vi "Main.vi"(11 "error in (no error)":errorcluster) -> (15 "error out":errorcluster)   [LabVIEW 2023]
uses:
  Controls/Operation.ctl
  Controls/State Cluster.ctl
  Controls/Main Data Cluster.ctl
  Controls/Sender Clone Cluster.ctl
  Controls/Receiver Clone Cluster.ctl
  Classes/Receiver/Receiver UI.vi
  Classes/Sender/Sender UI.vi
  Classes/Receiver/Receiver.lvclass
  Classes/Sender/Sender.lvclass
panel:
  in  "Receiver Clones":string(combo)
  in  "Sender Clones":string(combo)
  in  "Create Receiver Clone":bool
  in  "Create Sender Clone":bool
  in  "Load Receiver":bool
  in  "Load Sender":bool
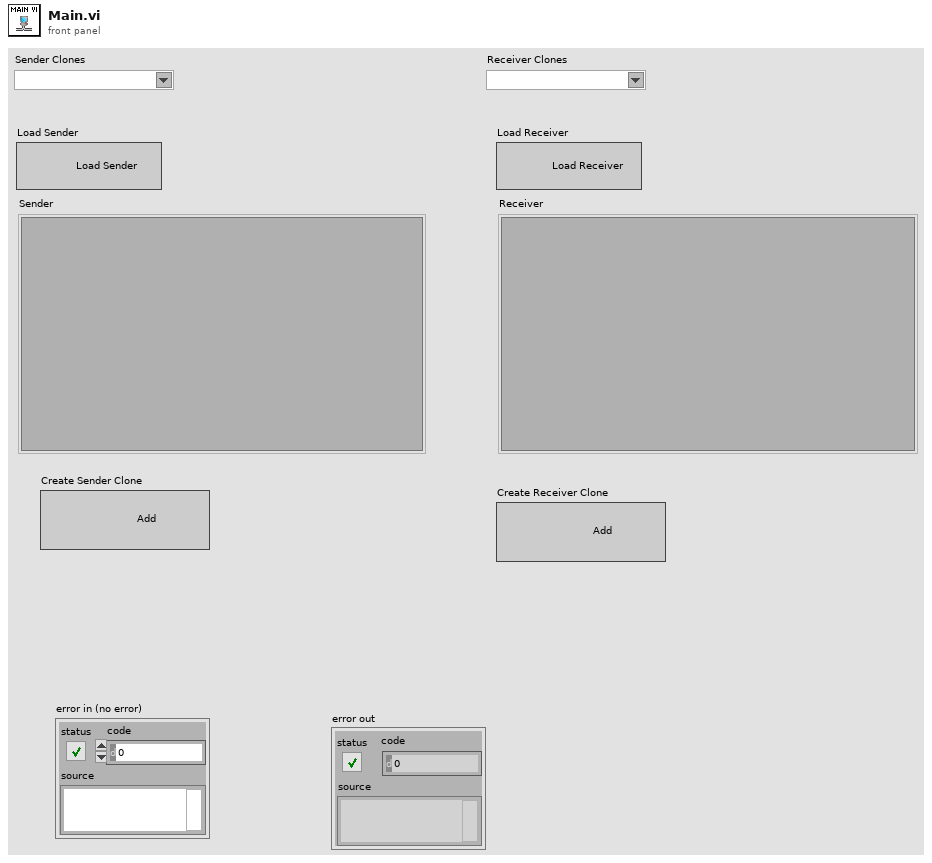
[diagram p1: front panel]
types:
  T1 = typedef "Main Data Cluster.ctl" = cluster{"user event out":refnum<user-event>, "Sender Path":path, "Receiver Path":path, "Sender Name":string, "Receiver Name":string, "Sender Combo Box":string[], "Sender Clone Data":T2[], "Receiver Clone Data":T3[], "Receiver Combo Box":string[], "Selected Receiver Clone":string, "Selected Sender Clone":string, "Sender VI Refnum":refnum<vi>, "Receiver VI Refnum":refnum<vi>, "Load/Unload Sender":bool, "Load/Unload Receiver":bool}
  T2 = typedef "Sender Clone Cluster.ctl" = cluster{"Sender Clone Name":string, "Sender VI reference":refnum<vi>}
  T3 = typedef "Receiver Clone Cluster.ctl" = cluster{"Receiver Clone Name":string, "Receiver VI Reference":refnum<vi>}
  T4 = typedef "State Cluster.ctl" = cluster{"State":string, "Data":variant}
  T5 = typedef "Operation.ctl" = enum16{"Create", "Enqueue", "Enqueue N", "Enstack", "Dequeue", "Flush", "Release"}
  T6 = enum8{"Enabled", "Disabled", "Disabled and Grayed Out"}
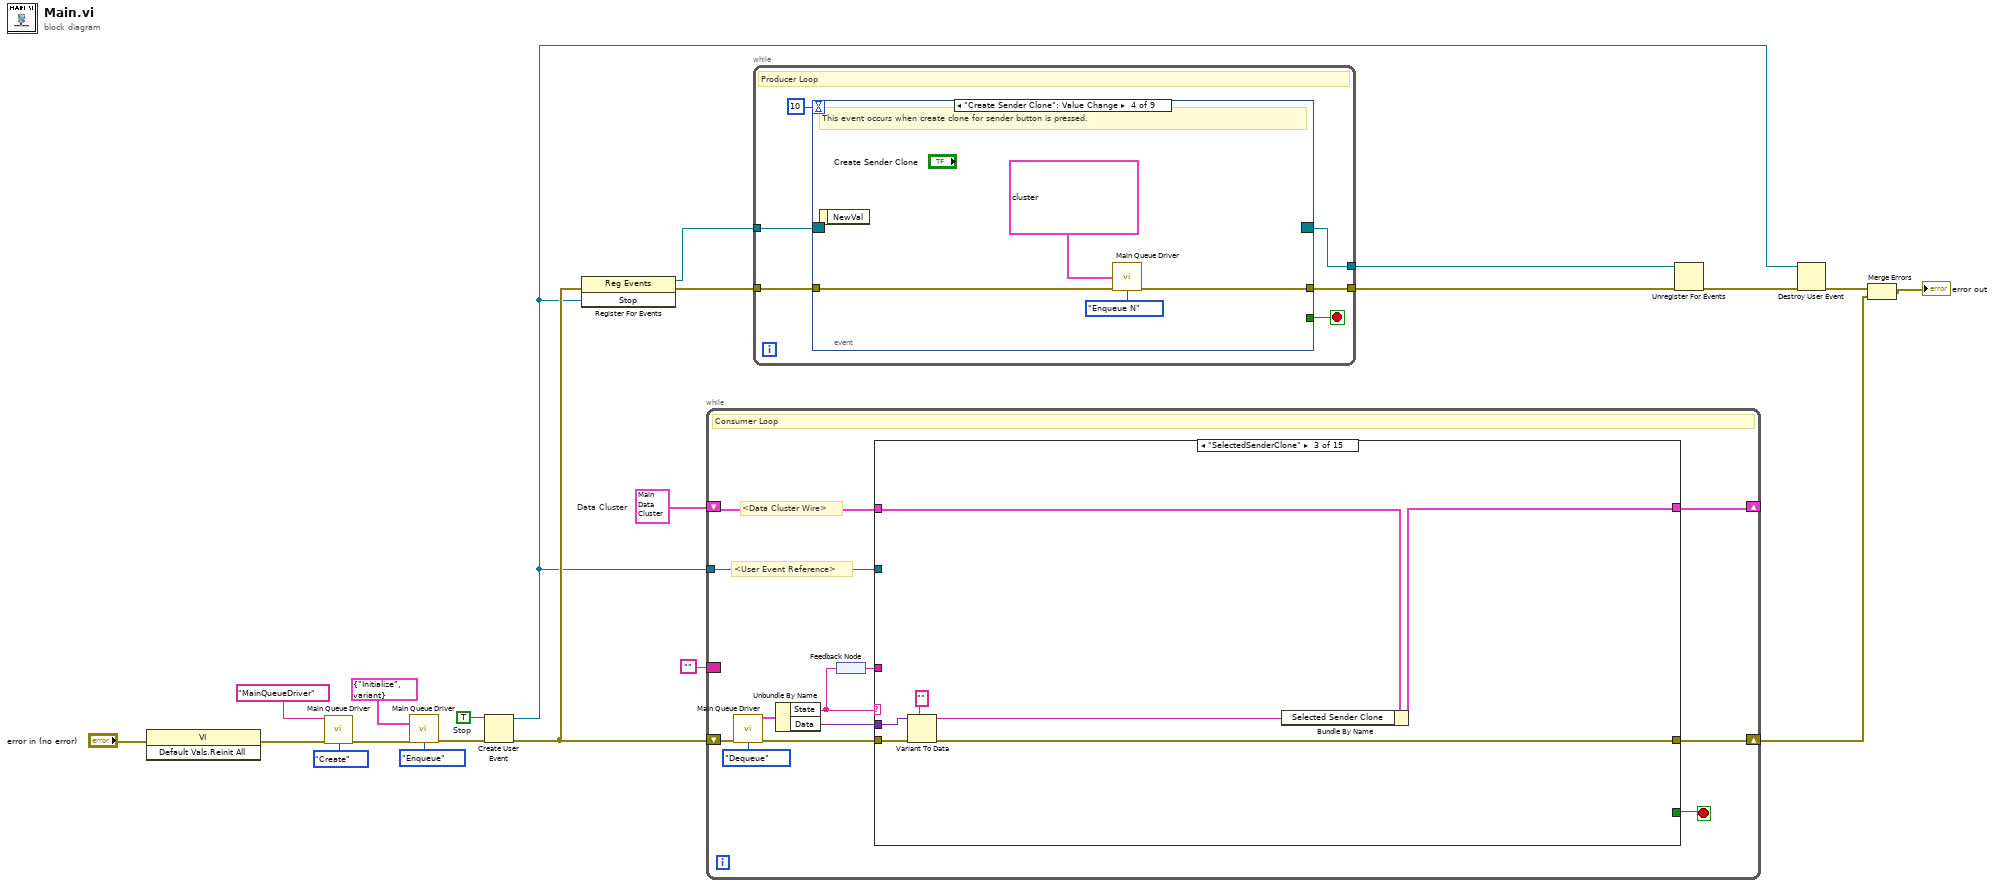
[diagram p0: block diagram]
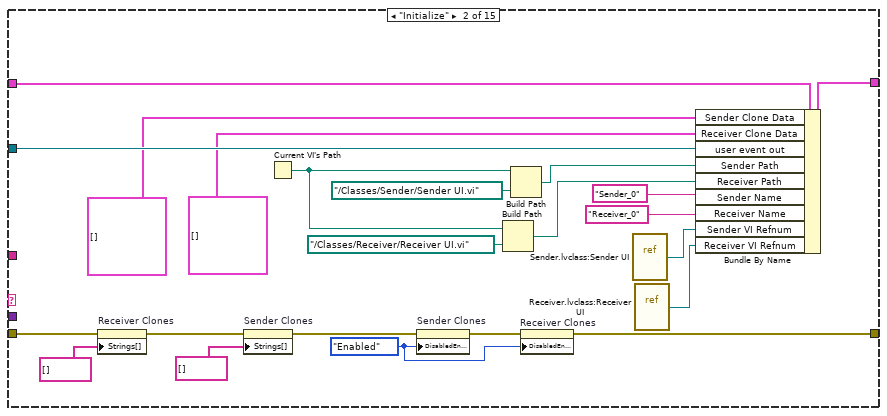
[diagram p3: hidden frame]
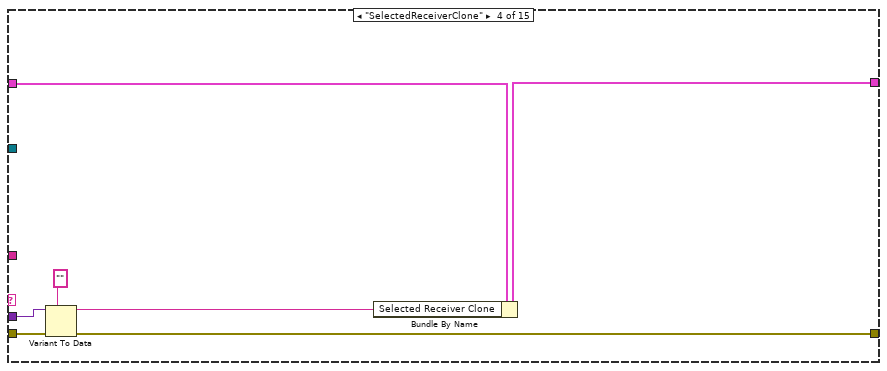
[diagram p4: hidden frame]
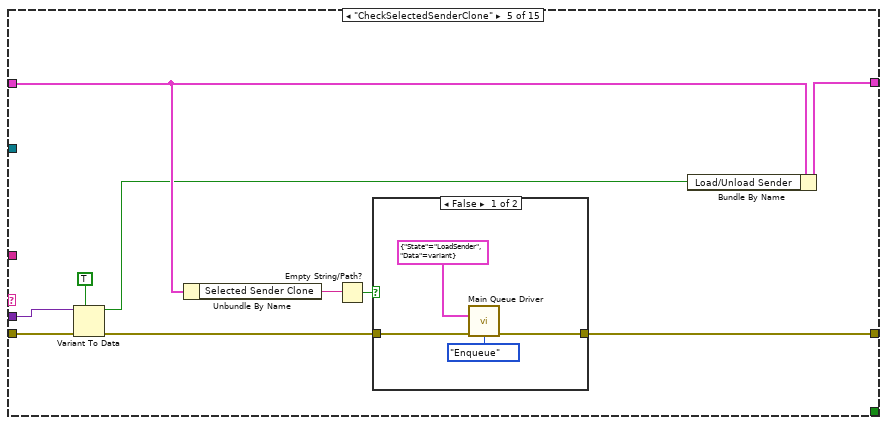
[diagram p5: hidden frame]
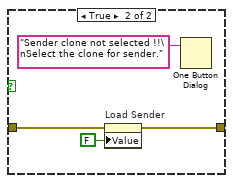
[diagram p6: hidden frame]
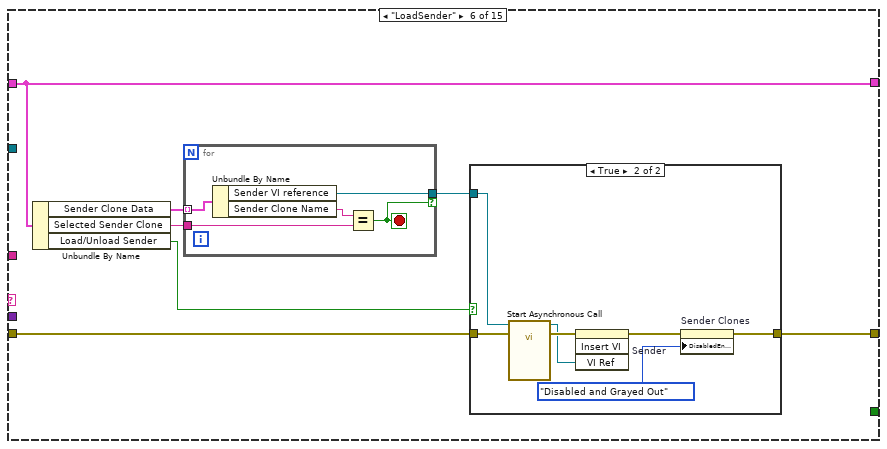
[diagram p7: hidden frame]
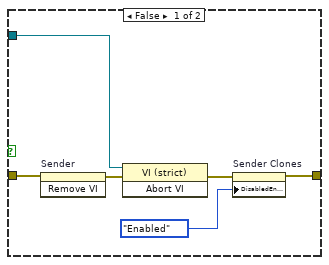
[diagram p8: hidden frame]
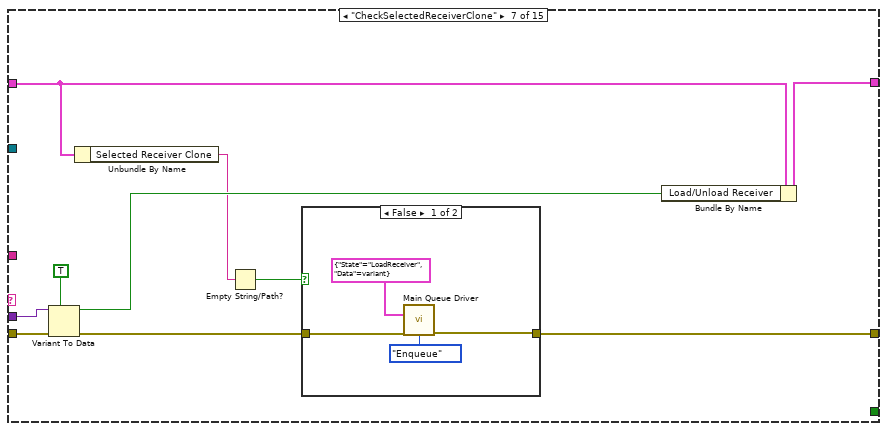
[diagram p9: hidden frame]
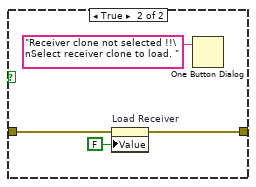
[diagram p10: hidden frame]
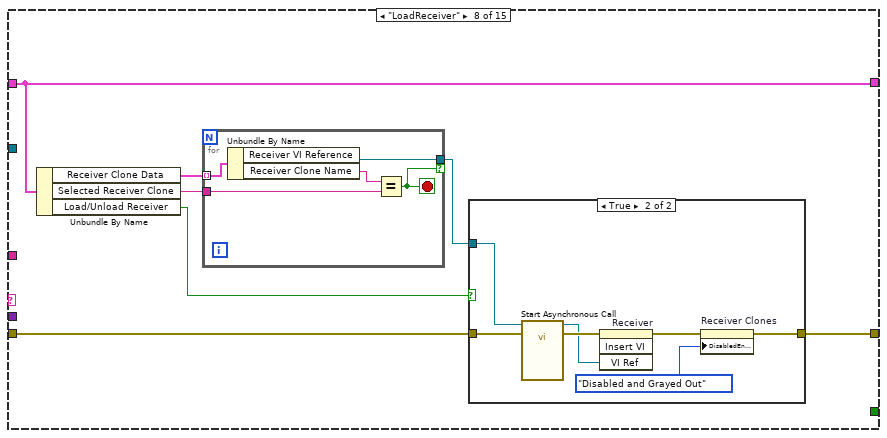
[diagram p11: hidden frame]
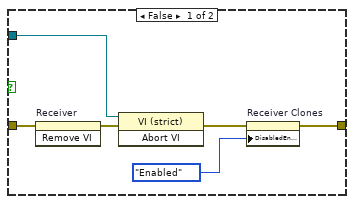
[diagram p12: hidden frame]
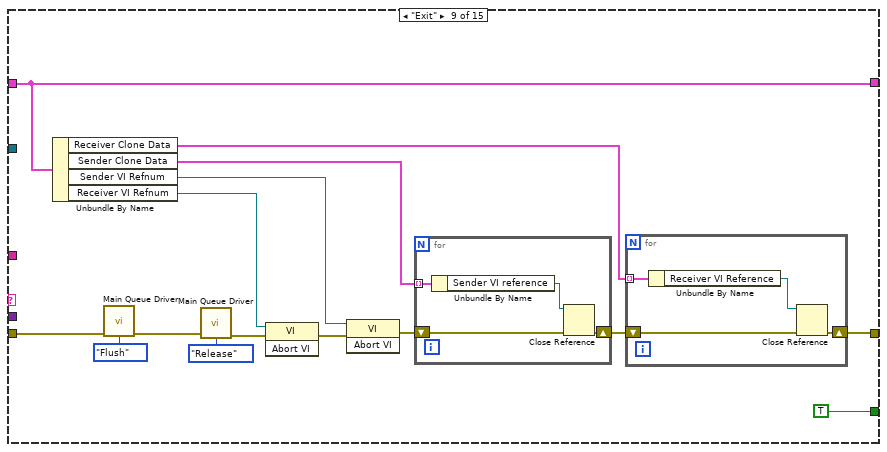
[diagram p13: hidden frame]
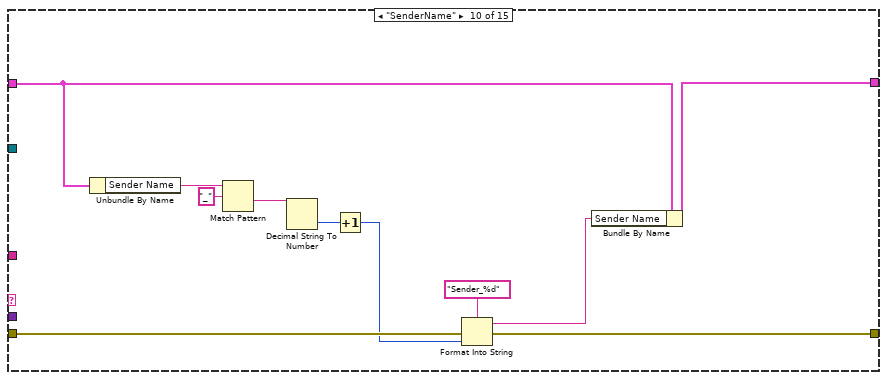
[diagram p14: hidden frame]
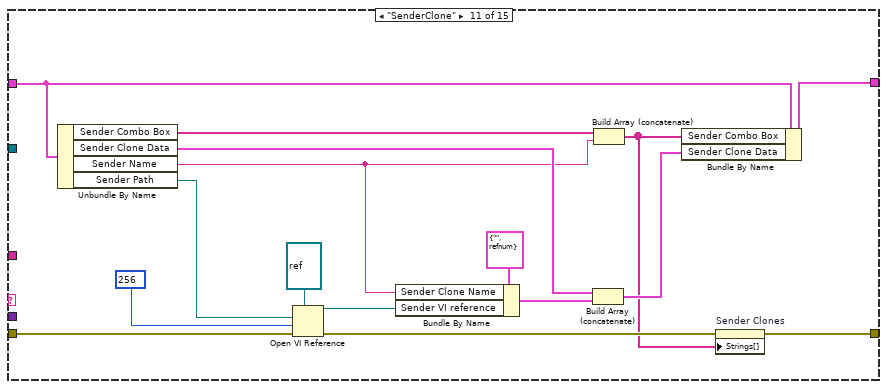
[diagram p15: hidden frame]
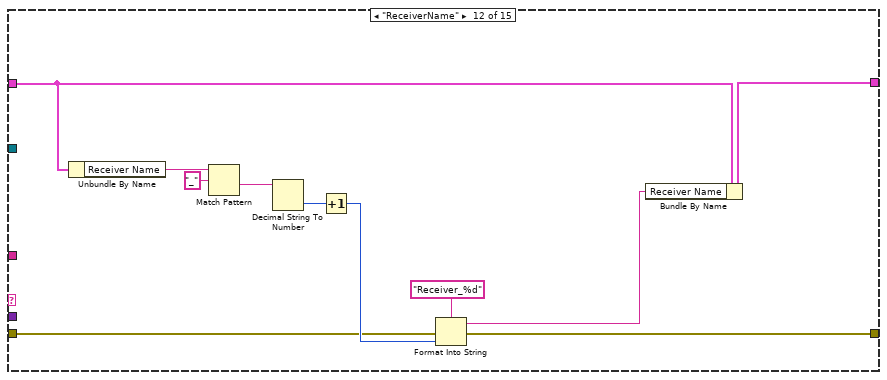
[diagram p16: hidden frame]
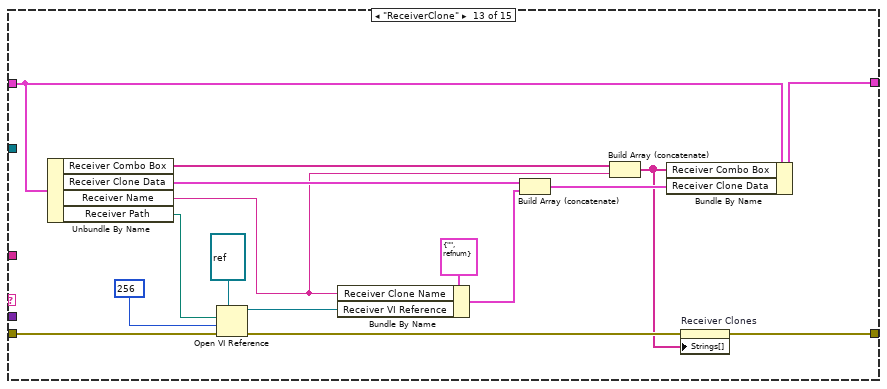
[diagram p17: hidden frame]
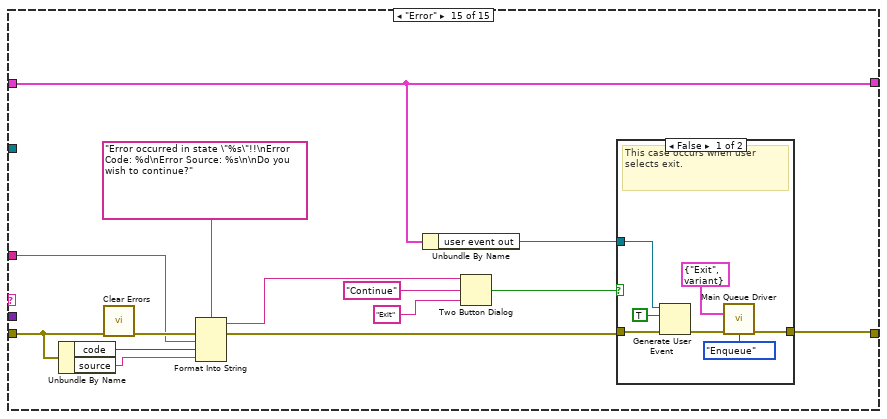
[diagram p19: hidden frame]
diagram:
  w4 = T1 {"user event out"=refnum, "Sender Path"=path "", "Receiver Path"=path "", "Sender Name"="", "Receiver Name"="", "Sender Combo Box"=[], "Sender Clone Data"=[], "Receiver Clone Data"=[], "Receiver Combo Box"=[], "Selected Receiver Clone"="", "Selected Sender Clone"="", "Sender VI Refnum"=refnum, "Receiver VI Refnum"=refnum, "Load/Unload Sender"=FALSE, "Load/Unload Receiver"=FALSE}  # Data Cluster
  w15 = TRUE  # Stop
  n1 = invoke class="VI" method="Default Vals.Reinit All"(error in="error in (no error)") -> (error out=w1:errorcluster)  [unwired: 2 in, 2 out]
  n2 = call "Main Queue Driver.vi"("Queue Name"="MainQueueDriver", "error in (no error)"=w1, "Operations"=Operation."Create") -> ("error out"=w19:errorcluster)  [unwired: 11 in, 1 out]
  n3 = call "Main Queue Driver.vi"("State"=T4 {"State"="Initialize", "Data"=variant}, "error in (no error)"=w19, "Operations"=Operation."Enqueue") -> ("error out"=w16:errorcluster)  [unwired: 11 in, 1 out]
  n4 = Create User Event(user event datatype=w15, error in=w16) -> (user event=w3:refnum<user-event>, error out=w14:errorcluster)
  n5 = register-events(error in=w14, w3) -> (reference out=w12:refnum<event-registration>, error out=w13:errorcluster)  [unwired: 1 in]
  n6 = while {
    shift-right: [w27] -> w6
    shift-left: w14 -> [w32]
    border: "" -> [_]
    tunnel: w3 -> [w24]
    shift-right: [w23] -> _
    shift-left: w4 -> [w25]
    stop <- w26 stop-if-true
    # "<User Event Reference>"
    # "<Data Cluster Wire>"
    # "Consumer Loop"
    n7 = call "Main Queue Driver.vi"("error in (no error)"=w32, "Operations"=Operation."Dequeue") -> ("Dequeued Element"=w30:T4, "error out"=w31:errorcluster)  [unwired: 12 in]
    n8 = Unbundle By Name(w30) -> ("State"=w28:string, "Data"=w29:variant)
    n9 = feedback-in #1(w28) -> ()
    n10 = feedback #1() -> (w22:string)
    n11 = case shown="\"SelectedSenderClone\"" w28 {
      tunnel: w31 -> [w35 w45 w64 w71 w81 w96 w124 w139 w171 w187 w205 w212 w231 w236 w243]
      tunnel: w29 -> [_ _ w62 w69 w80 _ w123 _ _ _ _ _ _ _ _]
      tunnel: [w35 w37 w63 w70 w72 w95 w115 w138 w159 w186 w195 w211 w221 w236 w240] -> w27
      tunnel: [_ _ _ _ _ _ _ _ TRUE _ _ _ _ _ _] -> w26
      tunnel: w25 -> [w34 w57 w60 w68 w77 w94 w119 w137 w166 w183 w204 w210 w230 w235 w239]
      tunnel: w24 -> [_ w56 _ _ _ _ _ _ _ _ _ _ _ _ _]
      tunnel: [w34 w55 w59 w67 w78 w94 w121 w137 w166 w182 w203 w209 w219 w235 w239] -> w23
      tunnel: w22 -> [_ _ _ _ _ _ _ _ _ _ _ _ _ _ w237]
      frame Default {
      }
      frame "Initialize" {
        w36 = T6."Enabled" ("Disabled")
        n12 = property on="Receiver Clones" class="CmbBox"(error in=w45, "Strings[]"=string[] [] ("Strings []")) -> (error out=w44:errorcluster)  [unwired: 1 in, 1 out]
        n13 = property on="Sender Clones" class="CmbBox"(error in=w44, "Strings[]"=string[] [] ("Strings []")) -> (error out=w39:errorcluster)  [unwired: 1 in, 1 out]
        n14 = Current VI's Path() -> (path=w51:path)
        n15 = property on="Sender Clones" class="CmbBox"(error in=w39, "DisabledEnum"=w36) -> (error out=w38:errorcluster)  [unwired: 1 in, 1 out]
        n16 = Build Path(base path=w51, name or relative path=path "../Classes/Receiver/Receiver UI.vi") -> (appended path=w50:path)
        n17 = Build Path(base path=w51, name or relative path=path "../Classes/Sender/Sender UI.vi") -> (appended path=w53:path)
        n18 = property on="Receiver Clones" class="CmbBox"(error in=w38, "DisabledEnum"=w36) -> (error out=w37:errorcluster)  [unwired: 1 in, 1 out]
        n19 = vi-ref "Sender.lvclass:Sender UI.vi"() -> (w41:refnum<vi>)
        n20 = vi-ref "Receiver.lvclass:Receiver UI.vi"() -> (w40:refnum<vi>)
        n21 = Bundle By Name(cluster=w57, "Sender Clone Data"=T2[] [], "Receiver Clone Data"=T3[] [], "user event out"=w56, "Sender Path"=w53, "Receiver Path"=w50, "Sender Name"="Sender_0", "Receiver Name"="Receiver_0", "Sender VI Refnum"=w41, "Receiver VI Refnum"=w40) -> (w55:T1)
      }
      frame "SelectedSenderClone" {
        n22 = Variant To Data(error in=w64, type="", Variant=w62) -> (data=w58:string, error out=w63:errorcluster)
        n23 = Bundle By Name(cluster=w60, "Selected Sender Clone"=w58) -> (w59:T1)
      }
      frame "SelectedReceiverClone" {
        n24 = Variant To Data(error in=w71, type="", Variant=w69) -> (data=w66:string, error out=w70:errorcluster)
        n25 = Bundle By Name(cluster=w68, "Selected Receiver Clone"=w66) -> (w67:T1)
      }
      frame "CheckSelectedSenderClone" {
        n26 = Variant To Data(error in=w81, type=TRUE, Variant=w80) -> (data=w73:bool, error out=w75:errorcluster)
        n27 = Unbundle By Name(w77) -> ("Selected Sender Clone"=w76:string)
        n28 = Empty String/Path?(string/path=w76) -> (empty?=w74:bool)
        n29 = case shown="False" w74 {
          tunnel: w75 -> [w85 w88]
          tunnel: [w84 w87] -> w72
          frame False {
            n30 = call "Main Queue Driver.vi"("State"=T4 {"State"="LoadSender", "Data"=variant}, "error in (no error)"=w85, "Operations"=Operation."Enqueue") -> ("error out"=w84:errorcluster)  [unwired: 11 in, 1 out]
          }
          frame True {
            n31 = property on="Load Sender" class="Bool (strict)"(error in=w88, "Value"=FALSE ("Load Sender")) -> (error out=w87:errorcluster)  [unwired: 1 in, 1 out]
            n32 = One Button Dialog(message="Sender clone not selected !!\nSelect the clone for sender.") -> ()  [unwired: 1 in, 1 out]
          }
        }
        n33 = Bundle By Name(cluster=w77, "Load/Unload Sender"=w73) -> (w78:T1)
      }
      frame "LoadSender" {
        n34 = Unbundle By Name(w94) -> ("Sender Clone Data"=w93:T2[], "Selected Sender Clone"=w92:string, "Load/Unload Sender"=w90:bool)
        n35 = for {
          tunnel: w93 -> [w101] mode=indexing
          tunnel: w92 -> [w99]
          tunnel: [w98] -> w91 if=w97
          stop <- w97 stop-if-true
          n36 = Unbundle By Name(w101) -> ("Sender VI reference"=w98:refnum<vi>, "Sender Clone Name"=w100:string)
          n37 = Equal?(x=w100, y=w99) -> (x = y?=w97:bool)
        }
        n38 = case shown="True" w90 {
          tunnel: [w103 w109] -> w95
          tunnel: w96 -> [w107 w114]
          tunnel: w91 -> [w105 w112]
          frame False {
            n39 = invoke on="Sender" class="SubPnl" method="Remove VI"(error in=w107) -> (error out=w106:errorcluster)  [unwired: 2 in, 2 out]
            n40 = invoke class="VI (strict)" method="Abort VI"(reference=w105, error in=w106) -> (error out=w104:errorcluster)  [unwired: 1 in, 2 out]
            n41 = property on="Sender Clones" class="CmbBox"(error in=w104, "DisabledEnum"=T6."Enabled" ("Disabled")) -> (error out=w103:errorcluster)  [unwired: 1 in, 1 out]
          }
          frame True {
            n42 = call-by-ref "Start Asynchronous Call"(reference=w112, error in=w114) -> (reference out=w111:refnum<vi>, error out=w113:errorcluster)  [unwired: 15 in, 1 out]
            n43 = invoke on="Sender" class="SubPnl" method="Insert VI"(error in=w113, "VI Ref"=w111) -> (error out=w110:errorcluster)  [unwired: 2 in, 3 out]
            n44 = property on="Sender Clones" class="CmbBox"(error in=w110, "DisabledEnum"=T6."Disabled and Grayed Out" ("Disabled")) -> (error out=w109:errorcluster)  [unwired: 1 in, 1 out]
          }
        }
      }
      frame "CheckSelectedReceiverClone" {
        n45 = Variant To Data(error in=w124, type=TRUE, Variant=w123) -> (data=w120:bool, error out=w116:errorcluster)
        n46 = Unbundle By Name(w119) -> ("Selected Receiver Clone"=w118:string)
        n47 = Empty String/Path?(string/path=w118) -> (empty?=w117:bool)
        n48 = case shown="False" w117 {
          tunnel: w116 -> [w128 w131]
          tunnel: [w127 w130] -> w115
          frame False {
            n49 = call "Main Queue Driver.vi"("State"=T4 {"State"="LoadReceiver", "Data"=variant}, "error in (no error)"=w128, "Operations"=Operation."Enqueue") -> ("error out"=w127:errorcluster)  [unwired: 11 in, 1 out]
          }
          frame True {
            n50 = property on="Load Receiver" class="Bool (strict)"(error in=w131, "Value"=FALSE ("Load Receiver")) -> (error out=w130:errorcluster)  [unwired: 1 in, 1 out]
            n51 = One Button Dialog(message="Receiver clone not selected !!\nSelect receiver clone to load. ") -> ()  [unwired: 1 in, 1 out]
          }
        }
        n52 = Bundle By Name(cluster=w119, "Load/Unload Receiver"=w120) -> (w121:T1)
      }
      frame "LoadReceiver" {
        n53 = Unbundle By Name(w137) -> ("Receiver Clone Data"=w136:T3[], "Selected Receiver Clone"=w135:string, "Load/Unload Receiver"=w133:bool)
        n54 = for {
          tunnel: w136 -> [w144] mode=indexing
          tunnel: w135 -> [w142]
          tunnel: [w141] -> w134 if=w140
          stop <- w140 stop-if-true
          n55 = Unbundle By Name(w144) -> ("Receiver VI Reference"=w141:refnum<vi>, "Receiver Clone Name"=w143:string)
          n56 = Equal?(x=w143, y=w142) -> (x = y?=w140:bool)
        }
        n57 = case shown="True" w133 {
          tunnel: [w146 w152] -> w138
          tunnel: w139 -> [w150 w157]
          tunnel: w134 -> [w148 w155]
          frame False {
            n58 = invoke on="Receiver" class="SubPnl" method="Remove VI"(error in=w150) -> (error out=w149:errorcluster)  [unwired: 2 in, 2 out]
            n59 = invoke class="VI (strict)" method="Abort VI"(reference=w148, error in=w149) -> (error out=w147:errorcluster)  [unwired: 1 in, 2 out]
            n60 = property on="Receiver Clones" class="CmbBox"(error in=w147, "DisabledEnum"=T6."Enabled" ("Disabled")) -> (error out=w146:errorcluster)  [unwired: 1 in, 1 out]
          }
          frame True {
            n61 = call-by-ref "Start Asynchronous Call"(reference=w155, error in=w157) -> (reference out=w154:refnum<vi>, error out=w156:errorcluster)  [unwired: 16 in]
            n62 = invoke on="Receiver" class="SubPnl" method="Insert VI"(error in=w156, "VI Ref"=w154) -> (error out=w153:errorcluster)  [unwired: 2 in, 3 out]
            n63 = property on="Receiver Clones" class="CmbBox"(error in=w153, "DisabledEnum"=T6."Disabled and Grayed Out" ("Disabled")) -> (error out=w152:errorcluster)  [unwired: 1 in, 1 out]
          }
        }
      }
      frame "Exit" {
        n64 = Unbundle By Name(w166) -> ("Receiver Clone Data"=w158:T3[], "Sender Clone Data"=w160:T2[], "Sender VI Refnum"=w163:refnum<vi>, "Receiver VI Refnum"=w162:refnum<vi>)
        n65 = call "Main Queue Driver.vi"("error in (no error)"=w171, "Operations"=Operation."Flush") -> ("error out"=w169:errorcluster)  [unwired: 12 in, 1 out]
        n66 = call "Main Queue Driver.vi"("error in (no error)"=w169, "Operations"=Operation."Release") -> ("error out"=w167:errorcluster)  [unwired: 12 in, 1 out]
        n67 = invoke class="VI" method="Abort VI"(reference=w162, error in=w167) -> (error out=w165:errorcluster)  [unwired: 1 in, 2 out]
        n68 = invoke class="VI" method="Abort VI"(reference=w163, error in=w165) -> (error out=w164:errorcluster)  [unwired: 1 in, 2 out]
        n69 = for {
          shift-right: [w179] -> w161
          shift-left: w164 -> [w180]
          tunnel: w160 -> [w178] mode=indexing
          n70 = Unbundle By Name(w178) -> ("Sender VI reference"=w177:refnum<vi>)
          n71 = Close Reference(reference=w177, error in (no error)=w180) -> (error out=w179:errorcluster)
        }
        n72 = for {
          shift-right: [w175] -> w159
          shift-left: w161 -> [w176]
          tunnel: w158 -> [w174] mode=indexing
          n73 = Unbundle By Name(w174) -> ("Receiver VI Reference"=w173:refnum<vi>)
          n74 = Close Reference(reference=w173, error in (no error)=w176) -> (error out=w175:errorcluster)
        }
      }
      frame "SenderName" {
        n75 = Unbundle By Name(w183) -> ("Sender Name"=w191:string)
        n76 = Match Pattern(string=w191, regular expression="_") -> (after substring=w189:string)  [unwired: 1 in, 3 out]
        n77 = Decimal String To Number(string=w189) -> (number=w188:i32)  [unwired: 2 in, 1 out]
        n78 = Increment(x=w188) -> (x+1=w185:i32)
        n79 = Format Into String(format string="Sender_%d", error in=w187, w185) -> (resulting string=w181:string, error out=w186:errorcluster)  [unwired: 1 in]
        n80 = Bundle By Name(cluster=w183, "Sender Name"=w181) -> (w182:T1)
      }
      frame "SenderClone" {
        n81 = Unbundle By Name(w204) -> ("Sender Combo Box"=w198:string[], "Sender Clone Data"=w201:T2[], "Sender Name"=w197:string, "Sender Path"=w206:path)
        n82 = Open VI Reference(type specifier VI Refnum (for type only)=refnum<vi> refnum, vi path=w206, options=256, error in (no error)=w205) -> (vi reference=w192:refnum<vi>, error out=w196:errorcluster)  [unwired: 2 in]
        n83 = Bundle By Name(cluster=T2 {"Sender Clone Name"="", "Sender VI reference"=refnum} ("Sender Clone"), "Sender Clone Name"=w197, "Sender VI reference"=w192) -> (w200:T2)
        n84 = Build Array (concatenate)(w201, w200) -> (w199:T2[])
        n85 = Build Array (concatenate)(w198, w197) -> (w194:string[])
        n86 = Bundle By Name(cluster=w204, "Sender Combo Box"=w194, "Sender Clone Data"=w199) -> (w203:T1)
        n87 = property on="Sender Clones" class="CmbBox"(error in=w196, "Strings[]"=w194) -> (error out=w195:errorcluster)  [unwired: 1 in, 1 out]
      }
      frame "ReceiverName" {
        n88 = Unbundle By Name(w210) -> ("Receiver Name"=w213:string)
        n89 = Match Pattern(string=w213, regular expression="_") -> (after substring=w216:string)  [unwired: 1 in, 3 out]
        n90 = Decimal String To Number(string=w216) -> (number=w217:i32)  [unwired: 2 in, 1 out]
        n91 = Increment(x=w217) -> (x+1=w218:i32)
        n92 = Format Into String(format string="Receiver_%d", error in=w212, w218) -> (resulting string=w208:string, error out=w211:errorcluster)  [unwired: 1 in]
        n93 = Bundle By Name(cluster=w210, "Receiver Name"=w208) -> (w209:T1)
      }
      frame "ReceiverClone" {
        n94 = Unbundle By Name(w230) -> ("Receiver Combo Box"=w224:string[], "Receiver Clone Data"=w227:T3[], "Receiver Name"=w223:string, "Receiver Path"=w233:path)
        n95 = Open VI Reference(type specifier VI Refnum (for type only)=refnum<vi> refnum, vi path=w233, options=256, error in (no error)=w231) -> (vi reference=w228:refnum<vi>, error out=w222:errorcluster)  [unwired: 2 in]
        n96 = Bundle By Name(cluster=T3 {"Receiver Clone Name"="", "Receiver VI Reference"=refnum}, "Receiver Clone Name"=w223, "Receiver VI Reference"=w228) -> (w226:T3)
        n97 = Build Array (concatenate)(w227, w226) -> (w225:T3[])
        n98 = Build Array (concatenate)(w224, w223) -> (w220:string[])
        n99 = Bundle By Name(cluster=w230, "Receiver Combo Box"=w220, "Receiver Clone Data"=w225) -> (w219:T1)
        n100 = property on="Receiver Clones" class="CmbBox"(error in=w222, "Strings[]"=w220) -> (error out=w221:errorcluster)  [unwired: 1 in, 1 out]
      }
      frame "FPUpdate" {
      }
      frame "Error" {
        n101 = Unbundle By Name(w243) -> ("code"=w242:i32, "source"=w241:string)
        n102 = call <vilib>:"Clear Errors.vi"("error in (no error)"=w243) -> ("error out"=w250:errorcluster)  [unwired: 5 in, 1 out]
        n103 = Format Into String(format string="Error occurred in state \"%s\"!!\nError Code: %d\nError Source: %s\n\nDo you wish to continue?", error in=w250, w237, w242, w241) -> (resulting string=w248:string, error out=w245:errorcluster)  [unwired: 1 in]
        n104 = Unbundle By Name(w239) -> ("user event out"=w238:refnum<user-event>)
        n105 = Two Button Dialog(message=w248, 1:"Exit" ("F button name (\"Cancel\")"), 2:"Continue" ("T button name (\"OK\")")) -> (T button?=w244:bool)
        n106 = case shown="False" w244 {
          tunnel: w245 -> [w257 w258]
          tunnel: [w253 w258] -> w240
          tunnel: w238 -> [w255 _]
          frame False {
            # "This case occurs when user selects exit."
            n107 = Generate User Event(user event=w255, event data cluster=TRUE ("event data"), error in=w257) -> (error out=w254:errorcluster)  [unwired: 1 in, 1 out]
            n108 = call "Main Queue Driver.vi"("State"=T4 {"State"="Exit", "Data"=variant}, "error in (no error)"=w254, "Operations"=Operation."Enqueue") -> ("error out"=w253:errorcluster)  [unwired: 11 in, 1 out]
          }
          frame True {
            # "This case occurs when user selects to continue."
          }
        }
      }
    }
  }
  n109 = while {
    tunnel: w13 -> [w263]
    tunnel: w12 -> [w262]
    tunnel: [w261] -> w10
    tunnel: [w260] -> w9
    stop <- w259 stop-if-true
    # "Producer Loop"
    n110 = event shown="[3] \"Create Sender Clone\": Value Change" {
      selector: w262 -> [_ _ _ _ _ _ _ _ _]
      dyn-events: [_ _ _ _ _ _ _ _ _] -> w261
      timeout: 10 -> [_ _ _ _ _ _ _ _ _]
      tunnel: w263 -> [w265 w269 w272 w276 w280 w287 w294 w301 w304]
      tunnel: [w265 w268 w272 w275 w279 w286 w293 w300 w303] -> w260
      tunnel: [_ w270 TRUE ("Discard?") _ _ _ _ _ _] -> w259
      event Timeout {
        # "This event occurs when no other event occurs."
        n111 = event-data() -> ()  [unwired: 1 in, 1 out]
      }
      event Panel Close? {
        w270 = TRUE ("Discard?")
        # "Occurs when panel close is pressed."
        n112 = event-data() -> ()  [unwired: 1 in, 1 out]
        n113 = call "Main Queue Driver.vi"("State"=T4 {"State"="Exit", "Data"=variant}, "error in (no error)"=w269, "Operations"=Operation."Enqueue") -> ("error out"=w268:errorcluster)  [unwired: 11 in, 1 out]
        n114 = event-data("Discard?"=w270) -> ()  [unwired: 1 in, 1 out]
      }
      event User Event {
        # "Occurs when stop user event is generated."
        n115 = event-data() -> ()  [unwired: 1 in, 1 out]
      }
      event "Create Sender Clone": Value Change {
        # "This event occurs when create clone for sender button is pressed."
        n116 = event-data() -> ()  [unwired: 1 in, 1 out]
        n117 = call "Main Queue Driver.vi"("State []"=T4[] [{"State"="SenderName", "Data"=variant}, {"State"="SenderClone", "Data"=variant}], "error in (no error)"=w276, "Operations"=Operation."Enqueue N") -> ("error out"=w275:errorcluster)  [unwired: 11 in, 1 out]
      }
      event "Create Receiver Clone": Value Change {
        # "This event occurs when user creates a new clone for receiver by pressing add button."
        n118 = event-data() -> ()  [unwired: 1 in, 1 out]
        n119 = call "Main Queue Driver.vi"("State []"=T4[] [{"State"="ReceiverName", "Data"=variant}, {"State"="ReceiverClone", "Data"=variant}], "error in (no error)"=w280, "Operations"=Operation."Enqueue N") -> ("error out"=w279:errorcluster)  [unwired: 11 in, 1 out]
      }
      event "Sender Clones": Value Change {
        # "This event occurs when user selects particular clone to load."
        n120 = event-data() -> ("NewVal"=w282:string)  [unwired: 1 in]
        n121 = To Variant(anything=w282) -> (Variant=w283:variant)
        n122 = Bundle By Name(cluster=T4 {"State"="SelectedSenderClone", "Data"=variant} ("State"), "Data"=w283) -> (w281:T4)
        n123 = call "Main Queue Driver.vi"("State"=w281, "error in (no error)"=w287, "Operations"=Operation."Enqueue") -> ("error out"=w286:errorcluster)  [unwired: 11 in, 1 out]
      }
      event "Receiver Clones": Value Change {
        # "This event occurs when user selects a clone for receiver."
        n124 = event-data() -> ("NewVal"=w289:string)  [unwired: 1 in]
        n125 = To Variant(anything=w289) -> (Variant=w290:variant)
        n126 = Bundle By Name(cluster=T4 {"State"="SelectedReceiverClone", "Data"=variant} ("State"), "Data"=w290) -> (w288:T4)
        n127 = call "Main Queue Driver.vi"("State"=w288, "error in (no error)"=w294, "Operations"=Operation."Enqueue") -> ("error out"=w293:errorcluster)  [unwired: 11 in, 1 out]
      }
      event "Load Sender": Value Change {
        # "This event occurs when load sender button is pressed."
        n128 = event-data() -> ()  [unwired: 1 in, 1 out]
        n129 = To Variant(anything="Load Sender") -> (Variant=w297:variant)
        n130 = Bundle By Name(cluster=T4 {"State"="CheckSelectedSenderClone", "Data"=variant} ("State"), "Data"=w297) -> (w295:T4)
        n131 = call "Main Queue Driver.vi"("State"=w295, "error in (no error)"=w301, "Operations"=Operation."Enqueue") -> ("error out"=w300:errorcluster)  [unwired: 11 in, 1 out]
      }
      event "Load Receiver": Value Change {
        # "This event occurs when load receiver button is pressed."
        n132 = event-data() -> ()  [unwired: 1 in, 1 out]
        n133 = To Variant(anything="Load Receiver") -> (Variant=w306:variant)
        n134 = Bundle By Name(cluster=T4 {"State"="CheckSelectedReceiverClone", "Data"=variant} ("State"), "Data"=w306) -> (w305:T4)
        n135 = call "Main Queue Driver.vi"("State"=w305, "error in (no error)"=w304, "Operations"=Operation."Enqueue") -> ("error out"=w303:errorcluster)  [unwired: 11 in, 1 out]
      }
    }
  }
  n136 = Unregister For Events(event registration refnum=w10, error in=w9) -> (error out=w8:errorcluster)
  n137 = Destroy User Event(user event=w3, error in=w8) -> (error out=w7:errorcluster)
  n138 = Merge Errors(w7, w6) -> (→"error out":errorcluster)
